vi "Generate Error Cluster.vi"(8 "error in (no error)":errorcluster, 9 "Additional Message":string, 10 "CallChainLvl (-1 => No call chain)":i32=1, 11 "Code":i32) -> (0 "error out":errorcluster)   [LabVIEW 2015, in "Data Replay File.lvlib"]
uses:
  Data Replay File.lvlib
panel:
  in  "VeriStand":string="NI VeriStand"
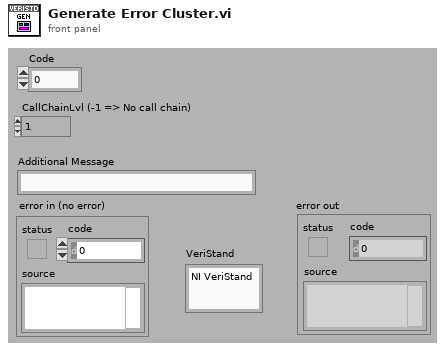
[diagram p1: front panel]
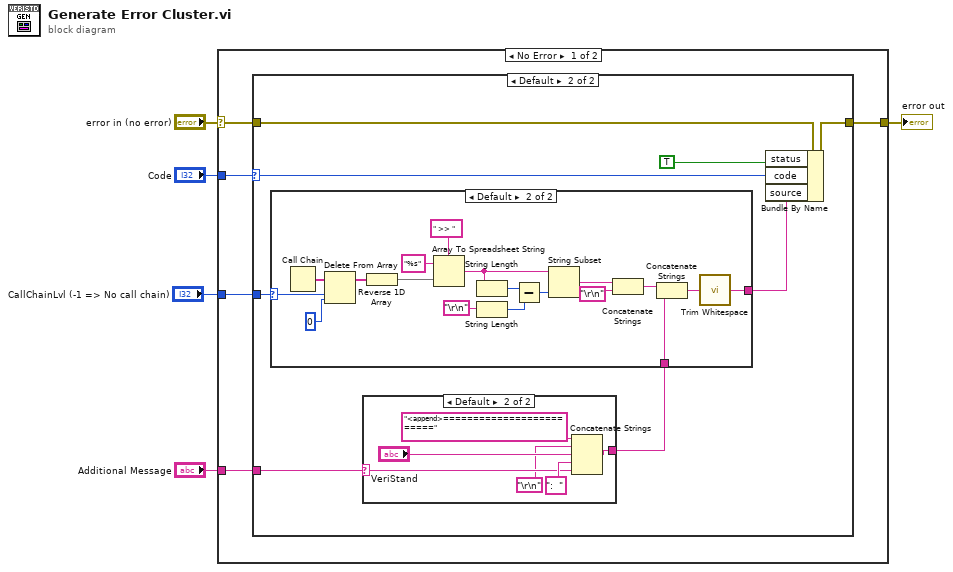
[diagram p0: block diagram]
diagram:
  n1 = case shown="No Error" "error in (no error)" {
    selector: "error in (no error)" -> [w7 w46]
    tunnel: [w10 w46] -> w4
    tunnel: "Code" -> [w6 _]
    tunnel: "Additional Message" -> [w9 _]
    tunnel: "CallChainLvl (-1 => No call chain)" -> [w8 _]
    frame No Error {
      n2 = case shown="Default" w6 {
        selector: w6 -> [_ w13]
        tunnel: [w11 w19] -> w10
        tunnel: w9 -> [_ w15]
        tunnel: w8 -> [_ w12]
        tunnel: w7 -> [w11 w14]
        frame 0 {
        }
        frame Default {
          n3 = case shown="Default" w15 {
            selector: w15 -> [w39 w42]
            tunnel: [w39 w43] -> w16
            frame "" {
            }
            frame Default {
              n4 = Concatenate Strings("<append>=========================", "\r\n", "VeriStand", ":  " ("string"), w42) -> (w43:string)
            }
          }
          n5 = case shown="Default" w12 {
            selector: w12 -> [_ w22]
            tunnel: [w20 w21] -> w17
            tunnel: w16 -> [w20 w35]
            frame ..-1 {
              # "No call chain"
            }
            frame Default {
              n6 = Call Chain() -> (call chain=w31:string[])
              n7 = Delete From Array(array=w31, length=w22, index=0 ("Index")) -> (array with subset deleted=w26:string[])  [unwired: 1 out]
              n8 = Reverse 1D Array(array=w26) -> (reversed array=w28:string[])
              n9 = Array To Spreadsheet String(delimiter (Tab)=" >> ", array=w28, 3:"%s" ("format string")) -> (spreadsheet string=w25:string)
              n10 = String Length(string=w25) -> (length=w29:i32)
              n11 = String Length(string="\r\n") -> (length=w23:i32)
              n12 = Subtract(x=w29, y=w23) -> (x-y=w30:i32)
              n13 = String Subset(string=w25, length (rest)=w30) -> (substring=w36:string)  [unwired: 1 out]
              n14 = Concatenate Strings(w36, "\r\n") -> (w37:string)
              n15 = Concatenate Strings(w37, w35) -> (w38:string)
              n16 = call <vilib>:"Trim Whitespace.vi"("string"=w38) -> ("trimmed string"=w21:string)  [unwired: 1 in]
            }
          }
          n17 = Bundle By Name(cluster=w14, "status"=TRUE, "code"=w13, "source"=w17) -> (w19:errorcluster)
        }
      }
    }
    frame Error {
      # "Cluster already contains error"
    }
  }
  "error out" <- w4
